vi "5 ch 1 sample resonance scanner (FPGA) fixed pix clock.vi"() -> ()   [LabVIEW 2012]
uses:
  <vilib>/eio/EIONode/EIONode.xnode
  <vilib>/rvi/eio/common/nirviEmuTemplateMethod_errors.vi
  <vilib>/rvi/DataTransferAndStorage/Container/XNode/niFpgaContainer.xnode
  <vilib>/rvi/interface/RandomDataEmulation/nirviRandomDataFpgaReadWriteTemplate.vi
  <vilib>/Platform/TimedLoop/XDataNode/XDataNode.xnode
  <vilib>/Platform/TimedLoop/XDataNode/nitl_modes.ctl
  <vilib>/Platform/TimedLoop/XDataNode/XDNodeRunTimeDep.lvlib
  <vilib>/Platform/TimedLoop/XDataNode/wakeup.ctl
  <vilib>/Platform/TimedLoop/XDataNode/timing_clust.ctl
panel:
  in  "lines at once":i16=4999
  in  "samples per half period":i16=4999
  in  "Start Delay (Ticks)":i16 caption="Start delay (Ticks)"
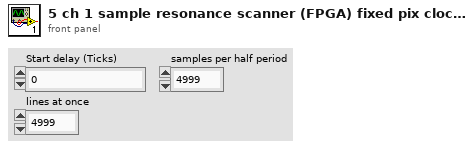
[diagram p1: front panel]
types:
  T1 = typedef "XDNodeRunTimeDep.lvlib/timing_clust.ctl" = cluster{"Expected End [f-1]":u64, "Actual End [f-1]":u64, "Finished Late? [f-1]":bool, "Expected End [i-1]":u64, "Actual End [i-1]":u64, "Finished Late? [i-1]":bool, "Expected Start [i]":u64, "Actual Start [i]":u64, "Expected Start [f]":u64, "Actual Start [f]":u64, "Source Name":string, "Structure Name":string, "Period":i64, "Deadline":i64, "Offset":i64, "Start":i64, "Priority":i32, "Timeout":i32, "Mode":T2, "Wakeup Reason":T3, "Error":errorcluster, "Source Type":string, "Secondary Source Type":string, "Global End Time":u64, "Global Start Time":u64, "Frame Duration":u64, "Iteration Duration":u64, "Assigned CPU":i32, "I/O Scan Engine Mode":u32}
  T2 = typedef "XDNodeRunTimeDep.lvlib/nitl_modes.ctl" = enum32{"No Change", "Process missed periods, maintain original phase", "Discard missed periods, maintain original phase", "Process missed periods, ignore original phase", "Discard missed periods, ignore original phase"}
  T3 = typedef "XDNodeRunTimeDep.lvlib/wakeup.ctl" = enum32{"Normal", "Aborted", "Asynchronous wakeup", "Timing source error", "Timed loop error", "Timeout"}
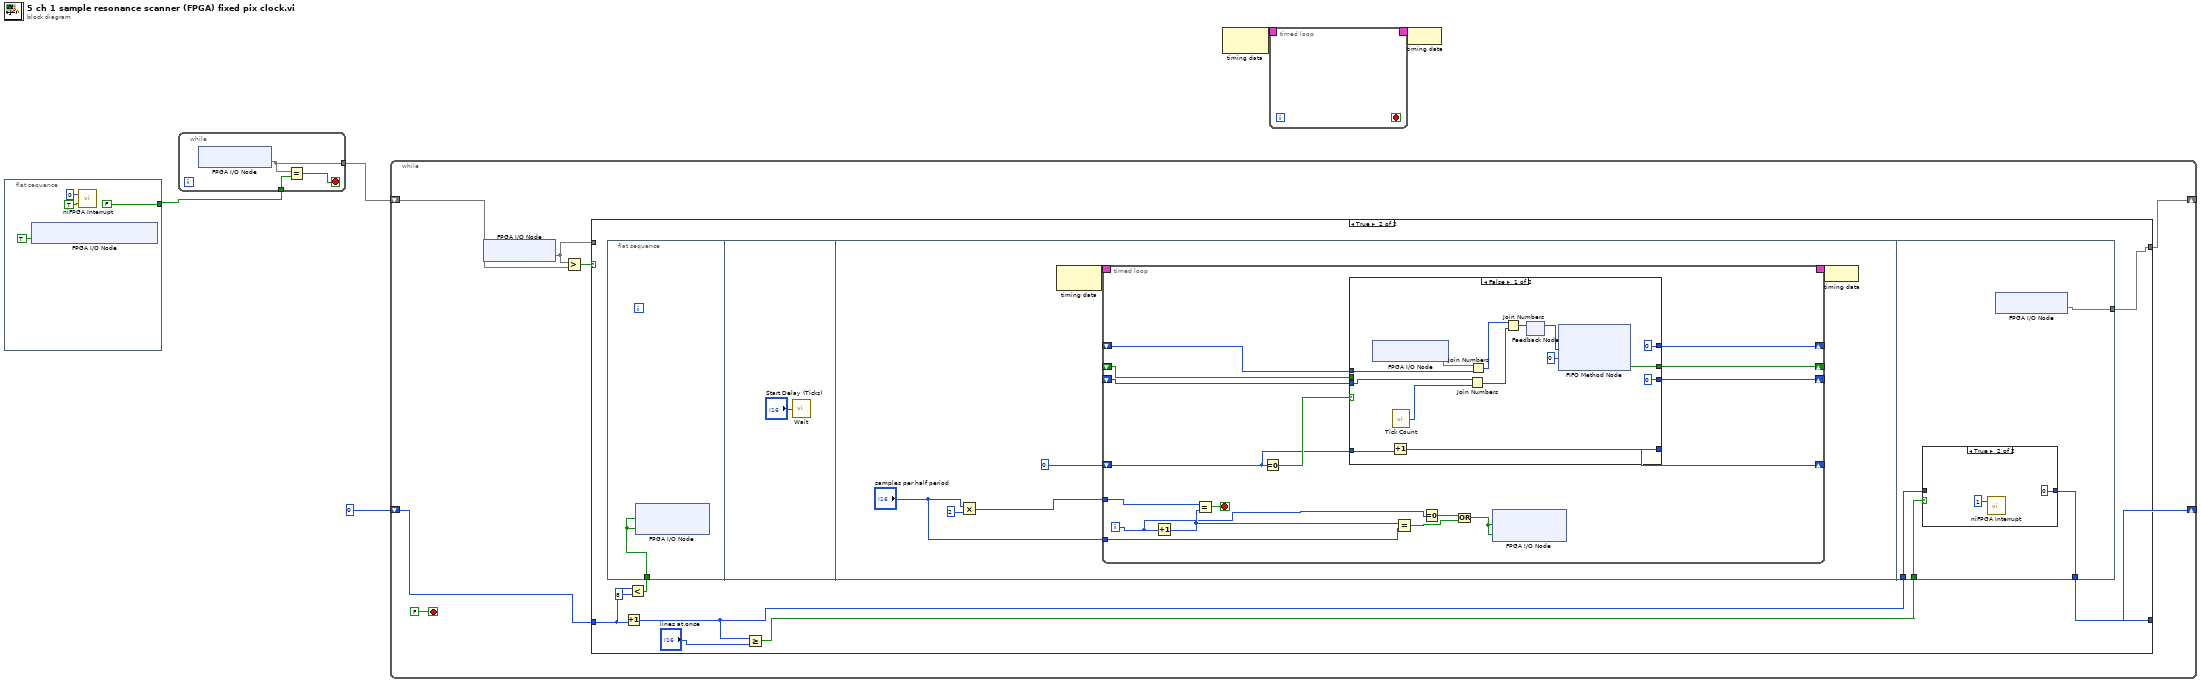
[diagram p0: block diagram]
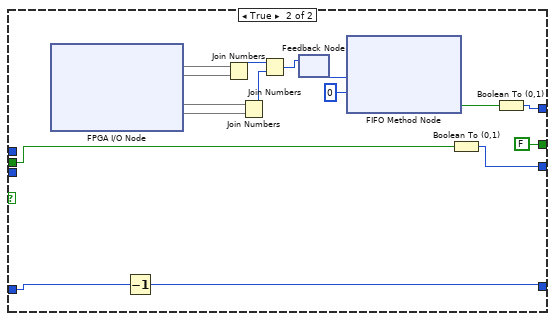
[diagram p3: hidden frame]
diagram:
  n1 = flat-sequence {
    tunnel: [FALSE ("IO Module\\DI 0")] -> w4
    frame #0 {
      n2 = xnode "FPGA I/O Node"("IO Module\\Digital Output Enable"=TRUE ("IO Module\\Digital Output Enable")) -> ()  [unwired: 1 in, 1 out]
      n3 = call <vilib>:"niFPGA Interrupt.vi"("Wait Until Cleared (F)"=TRUE, "IRQ Number (0)"=u8 0) -> ()  [unwired: 1 in]
    }
  }
  n4 = while {
    tunnel: w4 -> [w12]
    tunnel: [w10] -> w3
    stop <- w11 stop-if-true
    n5 = xnode "FPGA I/O Node"() -> ("IO Module\\DI 0"=w10)  [unwired: 1 in, 1 out]
    n6 = Equal?(x=w10, y=w12) -> (x = y?=w11:bool)
  }
  n7 = while {
    shift-right: [w18] -> _
    shift-left: w3 -> [w19]
    shift-right: [w16] -> _
    shift-left: i16 0 ("IRQ Number (0)") -> [w15]
    stop <- FALSE stop-if-true
    n8 = xnode "FPGA I/O Node"() -> ("IO Module\\DI 0"=w13)  [unwired: 1 in, 1 out]
    n9 = Greater?(x=w13, y=w19) -> (0:w14:bool)
    n10 = case shown="True" w14 {
      tunnel: [w20 w22] -> w18
      tunnel: w15 -> [w21 w25]
      tunnel: [w21 w27] -> w16
      tunnel: w13 -> [w20 _]
      frame False {
      }
      frame True {
        n11 = flat-sequence {
          tunnel: w23 -> [w30]
          tunnel: w29 -> [w92]
          tunnel: w28 -> [w91]
          tunnel: [w90] -> w27
          tunnel: [w89] -> w22
          frame #0 {
            n12 = xnode "FPGA I/O Node"("PXI_Trig2"=w30, "IO Module\\D0 2"=w30) -> ()  [unwired: 2 in, 2 out]
          }
          frame #1 {
            n13 = call "Wait"("Count(Ticks)"="Start Delay (Ticks)") -> ()  [unwired: 1 out]
          }
          frame #2 {
            n14 = Multiply(x="samples per half period", y=i16 2) -> (x*y=w36:i16)
            n15 = node-c288() -> (w35:T1)  [unwired: 1 in]
            n16 = timed-loop {
              tunnel: w36 -> [w53]
              timing: w35 -> [_]
              timing-out: [_] -> w34
              shift-right: [w50] -> _
              shift-left: 0 ("Timeout") -> [w51]
              shift-right: [w49] -> _
              shift-left: _ -> [w48]
              shift-right: [w47] -> _
              shift-left: _ -> [w44]
              shift-right: [w46] -> _
              shift-left: _ -> [w45]
              tunnel: "samples per half period" -> [w39]
              i -> [w38]
              stop <- w54 stop-if-true
              n17 = Increment(x=w38) -> (x+1=w40:i32)
              n18 = Equal?(x=w53, y=w40) -> (x = y?=w54:bool)
              n19 = Equal To 0?(x=w51) -> (x = 0?=w52:bool)
              n20 = case shown="False" w52 {
                tunnel: w51 -> [w68 w82]
                tunnel: [w67 w81] -> w50
                tunnel: [w61 FALSE ("Timed Out?")] -> w49
                tunnel: w48 -> [_ w73]
                tunnel: [i16 0 w72] -> w47
                tunnel: [i16 0 w71] -> w46
                tunnel: w45 -> [w60 _]
                tunnel: w44 -> [w59 _]
                frame False {
                  n21 = xnode "FPGA I/O Node"() -> ("IO Module\\AI B8"=w64)  [unwired: 1 in, 1 out]
                  n22 = Increment(x=w68) -> (x+1=w67:i32)
                  n23 = call "Tick Count"() -> ("Tick Count(Ticks)"=w58:u32)
                  n24 = Join Numbers(hi=w60, lo=w58) -> ((hi.lo)=w62:u64)
                  n25 = Join Numbers(hi=w64, lo=w59) -> ((hi.lo)=w63:u32)
                  n26 = Join Numbers(hi=w63, lo=w62) -> ((hi.lo)=w65:u64)
                  n27 = feedback-in #1(w65) -> ()
                  n28 = feedback #1() -> (w55:u64)  [unwired: 1 in]
                  n29 = xnode ("FIFO Method Node")("Element"=w55, "Timeout"=0) -> ("Timed Out?"=w61:bool)  [unwired: 1 in, 1 out]
                }
                frame True {
                  n30 = xnode "FPGA I/O Node"() -> ("IO Module\\AI A0"=w77, "IO Module\\AI A1"=w78, "IO Module\\AI A3"=w79, "IO Module\\AI A6"=w80)  [unwired: 4 in, 4 out]
                  n31 = Decrement(x=w82) -> (x-1=w81:i32)
                  n32 = Join Numbers(hi=w77, lo=w78) -> ((hi.lo)=w76:u32)
                  n33 = Join Numbers(hi=w79, lo=w80) -> ((hi.lo)=w75:u32)
                  n34 = Join Numbers(hi=w76, lo=w75) -> ((hi.lo)=w84:u64)
                  n35 = feedback-in #2(w84) -> ()
                  n36 = feedback #2() -> (w69:u64)  [unwired: 1 in]
                  n37 = xnode ("FIFO Method Node")("Element"=w69, "Timeout"=0) -> ("Timed Out?"=w74:bool)  [unwired: 1 in, 1 out]
                  n38 = Boolean To (0,1)(Boolean=w73) -> (0, 1=w71:i16)
                  n39 = Boolean To (0,1)(Boolean=w74) -> (0, 1=w72:i16)
                }
              }
              n40 = Equal?(x=w40, y=w39) -> (x = y?=w42:bool)
              n41 = Equal To 0?(x=w38) -> (x = 0?=w43:bool)
              n42 = Or(x=w43, y=w42) -> (x .or. y?=w41:bool)
              n43 = xnode "FPGA I/O Node"("IO Module\\D0 1"=w41, "PXI_Trig1"=w41) -> ()  [unwired: 2 in, 2 out]
            }
            n44 = node-c288(w34) -> ()
          }
          frame #3 {
            n45 = case shown="True" w91 {
              tunnel: w92 -> [w93 _]
              tunnel: [w93 u8 0] -> w90
              frame False {
              }
              frame True {
                n46 = call <vilib>:"niFPGA Interrupt.vi"("IRQ Number (0)"=u8 1) -> ()  [unwired: 2 in]
              }
            }
            n47 = xnode "FPGA I/O Node"() -> ("IO Module\\DI 0"=w89)  [unwired: 1 in, 1 out]
          }
        }
        n48 = Increment(x=w25) -> (x+1=w29:i16)
        n49 = Less?(x=w25, y=i16 8) -> (x < y?=w23:bool)
        n50 = Greater Or Equal?(x=w29, y="lines at once") -> (x >= y?=w28:bool)
      }
    }
  }
  n51 = node-c288() -> (w2:T1)  [unwired: 1 in]
  n52 = timed-loop {
    timing: w2 -> [_]
    timing-out: [_] -> w1
    stop <- _ stop-if-true
  }
  n53 = node-c288(w1) -> ()
